vi "gentec-M-Link.Open Connection.vi"(0 "VISA resource (In)":refnum<visa-resource-name>, 5 "error in (no error)":errorcluster) -> (14 "VISA resource (Out)":refnum<visa-resource-name>, 19 "error out":errorcluster)   [LabVIEW 2014, in "gentec-M-Link - Driver.lvlib"]
doc: "This VI opens a VISA connection and sets several attributes."
uses:
  gentec-M-Link - Driver.lvlib
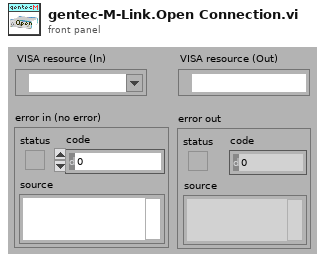
[diagram p1: front panel]
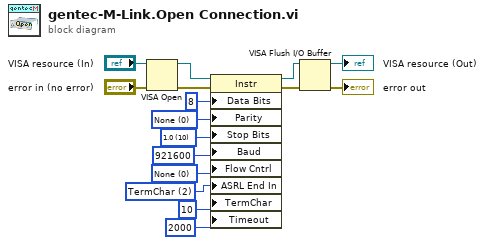
[diagram p0: block diagram]
diagram:
  w7 = u16 2 items=["None", "Last Bit", "TermChar", "Break"] ("Serial Settings:End Mode for Writes")
  w8 = u16 0 items=["None", "XON/XOFF", "RTS/CTS", "XON/XOFF & RTS/CTS", "DTR/DSR", "XON/XOFF & DTR/DSR"] ("Serial Settings:Flow Control")
  w10 = u16 10 items=["1.0"=10, "1.5"=15, "2.0"=20] ("Serial Settings:Stop Bits")
  w11 = u16 0 items=["None", "Odd", "Even", "Mark", "Space"] ("Serial Settings:Parity")
  n1 = VISA Open(error in (no error)="error in (no error)", VISA resource name="VISA resource (In)") -> (VISA resource name=w14:refnum<visa-resource-name>, error out=w13:errorcluster)  [unwired: 3 in]
  n2 = property class="Instr"(reference=w14, error in=w13, "Data Bits"=u16 8 ("Serial Settings:Data Bits"), "Parity"=w11, "Stop Bits"=w10, "Baud"=u32 921600 ("Serial Settings:Baud Rate"), "Flow Cntrl"=w8, "ASRL End In"=w7, "TermChar"=u8 10 ("Message Based Settings:Termination Character"), "Timeout"=u32 2000 ("General Settings:Timeout Value")) -> (reference out=w5:refnum<visa-resource-name>, error out=w4:errorcluster)
  n3 = VISA Flush I/O Buffer(VISA resource name=w5, error in (no error)=w4) -> (VISA resource name out=→"VISA resource (Out)":refnum<visa-resource-name>, error out=→"error out":errorcluster)  [unwired: 1 in]
